vi "Temperature Limit.vi"() -> ()   [LabVIEW 2015]
doc: "This VI simulates the acquisition of temperature, graphs the temperature, and notifies the user if the temperature is over the limit."
uses:
  <vilib>/Utility/miscctls.llb/LVPositionTypeDef.ctl
panel:
  in  "Start":bool
  in  "Delta t (ms)":i32(slide)=400 scale=50.0..500.0
  in  "Stop":bool
  in  "High Limit":dbl=28.0 format="%.2f"
  out "Temperature":cluster{"Temperature":dbl, "High Limit":dbl}(graph)={"Temperature"=85.88749999999999, "High Limit"=80.0}
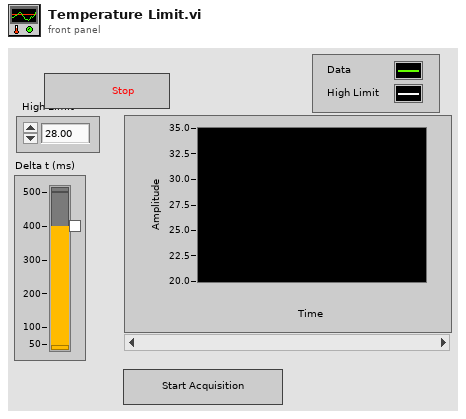
[diagram p1: front panel]
types:
  T1 = enum8{"Enabled", "Disabled", "Disabled and Grayed Out"}
  T2 = enum16{"Always On", "Always Off", "Off While Running"}
  T3 = typedef "LVPositionTypeDef.ctl" = cluster{"Left":i32, "Top":i32}
  T4 = cluster{"Temperature Value":dbl, "High Limit":dbl}
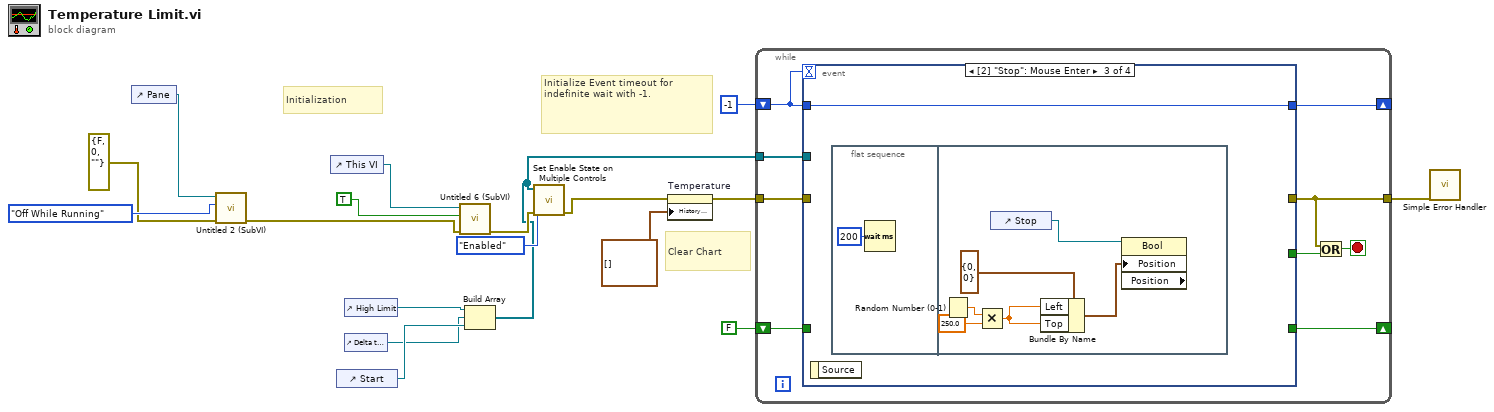
[diagram p0: block diagram]
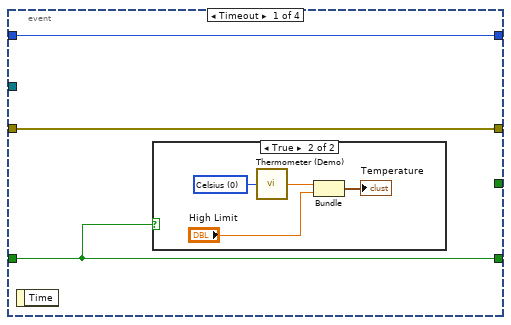
[diagram p2: hidden frame]
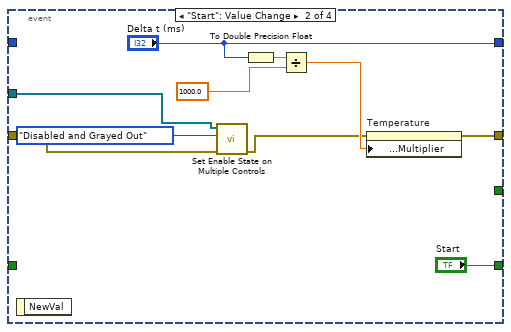
[diagram p4: hidden frame]
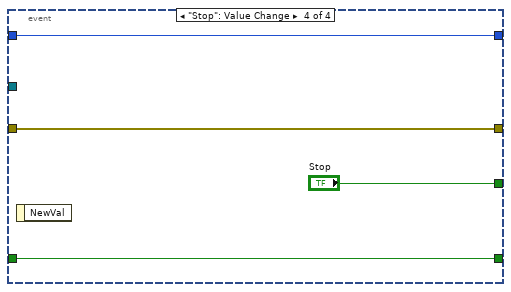
[diagram p5: hidden frame]
diagram:
  # "Clear Chart"
  # "Initialize Event timeout for indefinite wait with -1."
  # "Initialization"
  n1 = control-ref of="Pane"() -> (w11:refnum<vi>)
  n2 = call "Untitled 2 (SubVI).vi"("error in (no error)"=errorcluster {"status"=FALSE, "code"=0, "source"=""}, "Horizontal Scrollbar Visibility"=T2."Off While Running", "Pane in"=w11) -> ("error out"=w8:errorcluster)  [unwired: 7 in, 1 out]
  n3 = control-ref of="This VI"() -> (w9:refnum<vi>)
  n4 = control-ref of="Start"() -> (w3:refnum<vi>)
  n5 = control-ref of="High Limit"() -> (w1:refnum<vi>)
  n6 = control-ref of="Delta t (ms)"() -> (w2:refnum<vi>)
  n7 = call "Untitled 6 (SubVI).vi"("error in (no error)"=w8, "Boolean"=TRUE, "VI in"=w9) -> ("error out"=w6:errorcluster)  [unwired: 7 in, 1 out]
  n8 = Build Array(w1, w2, w3) -> (w4:refnum<vi>[])
  n9 = call "Set Enable State on Multiple Controls.vi"("Error In"=w6, "Disabled State"=T1."Enabled", "Controls"=w4) -> ("Error Out"=w7:errorcluster)  [unwired: 8 in]
  n10 = property on="Temperature" class="WFChart (strict)"(error in=w7, "History Data"=cluster{"Temperature":dbl, "High Limit":dbl}[] []) -> (error out=w17:errorcluster)  [unwired: 1 in, 1 out]
  n11 = while {
    tunnel: w17 -> [w27]
    tunnel: [w25] -> w15
    shift-right: [w23] -> _
    shift-left: FALSE ("Start") -> [w22]
    shift-right: [w21] -> _
    shift-left: -1 ("Delta t (ms)") -> [w20]
    tunnel: w4 -> [w19]
    stop <- w26 stop-if-true
    n12 = event shown="[2] \"Stop\": Mouse Enter" {
      selector: _ -> [_ _ _ _]
      dyn-events: _ -> [_ _ _ _]
      timeout: w20 -> [_ _ _ _]
      tunnel: [_ _ _ "Stop"] -> w24
      tunnel: w27 -> [w30 w38 _ w55]
      tunnel: [w30 w44 _ w55] -> w25
      tunnel: [w28 "Start" _ w54] -> w23
      tunnel: w22 -> [w28 _ _ w54]
      tunnel: [w29 "Delta t (ms)" w45 w53] -> w21
      tunnel: w20 -> [w29 _ w45 w53]
      tunnel: w19 -> [_ w35 _ _]
      event Timeout {
        n13 = event-data() -> ()  [unwired: 1 in, 1 out]
        n14 = case shown="True" w28 {
          frame False {
          }
          frame True {
            w31 = u16 0 items=["Celsius", "Fahrenheit"] ("Units (0: Celsius)")
            n15 = call "Thermometer (Demo).vi"("Units (0: Celsius)"=w31) -> ("Temperature Value"=w32:dbl)
            n16 = Bundle("Temperature Value"=w32, "High Limit"="High Limit") -> (→"Temperature":T4)  [unwired: 1 in]
          }
        }
      }
      event "Start": Value Change {
        n17 = event-data() -> ()  [unwired: 1 in, 1 out]
        n18 = call "Set Enable State on Multiple Controls.vi"("Error In"=w38, "Disabled State"=T1."Disabled and Grayed Out", "Controls"=w35) -> ("Error Out"=w37:errorcluster)  [unwired: 8 in]
        n19 = To Double Precision Float(number="Delta t (ms)") -> (double precision float=w43:dbl)
        n20 = Divide(x=w43, y=1000.0) -> (x/y=w41:dbl)
        n21 = property on="Temperature" class="WFChart (strict)"(error in=w37, "X Scale.Offset and Multiplier:Multiplier"=w41) -> (error out=w44:errorcluster)  [unwired: 1 in, 1 out]
      }
      event "Stop": Mouse Enter {
        n22 = event-data() -> ()  [unwired: 1 in, 1 out]
        n23 = flat-sequence {
          frame #0 {
            n24 = Wait (ms)(milliseconds to wait=u32 200) -> ()  [unwired: 1 out]
          }
          frame #1 {
            n25 = Random Number (0-1)() -> (number: 0 to 1=w49:dbl)
            n26 = Multiply(x=w49, y=250.0) -> (x*y=w47:dbl)
            n27 = control-ref of="Stop"() -> (w52:refnum<vi>)
            n28 = Bundle By Name(cluster=T3 {"Left"=0, "Top"=0} ("Position"), "Left"=w47, "Top"=w47) -> (w50:T3)
            n29 = property class="Bool" props=["Position", "Position"](reference=w52, "Position"=w50) -> ()  [unwired: 1 in, 3 out]
          }
        }
      }
      event "Stop": Value Change {
        n30 = event-data() -> ()  [unwired: 1 in, 1 out]
      }
    }
    n31 = Or(x=w25, y=w24) -> (x .or. y?=w26:bool)
  }
  n32 = call <vilib>:"Simple Error Handler.vi"("error in (no error)"=w15) -> ()  [unwired: 4 in, 5 out]
